vi "Ocean Optics 2000 4000 Process Spectrum.vi"() -> ()   [LabVIEW 2021]
doc: "Demonstrates measuring and processing the spectra and display in Absorbance, Transmission and Irradiance mode.\n\n<b>Note:</b>\nRefer to Spectrum Processing.vi for more details regarding the modes."
uses:
  <instrlib>/Ocean Optics 2000 4000/Ocean Optics 2000 4000.lvlib
panel:
  in  "Stop":bool
  out "Waveform":T1(graph)
  in  "Color Temperature (2850 K)":dbl=2850.0
  in  "Spectral Mode (0:Absorbance)":u16(ring) items=["Absorbance", "Transmission", "Irradiance"]
  in  "Read Reference":bool
  in  "Read Dark":bool
  in  "VISA resource name":refnum<visa-resource-name>
  # "(c) 2009-2016 National Instruments.  ALL RIGHTS RESERVED."
  # "To run this Example, select the spectral processing mode. Then run the VI. To read the dark spectrum, click Read Dark. Then click Read Reference to read Reference Spectrum. The processed spectrum will display on the graph. Press Stop when done."
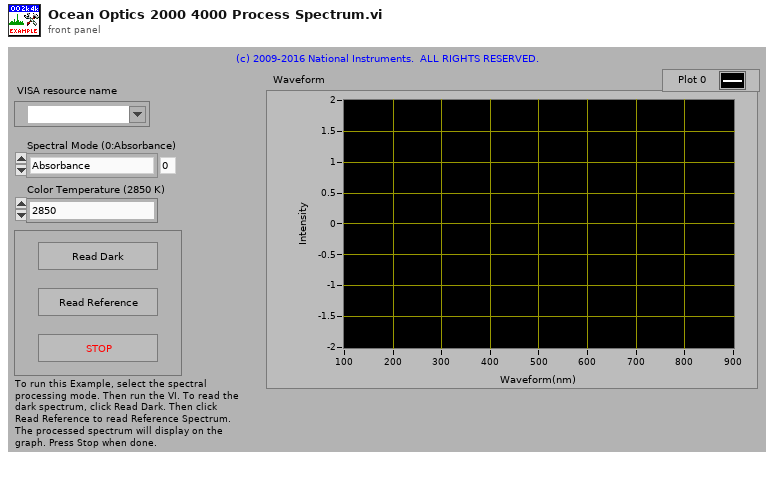
[diagram p1: front panel]
types:
  T1 = cluster{"Wavelength (nm)":dbl[], "Processed Spectrum":dbl[]}
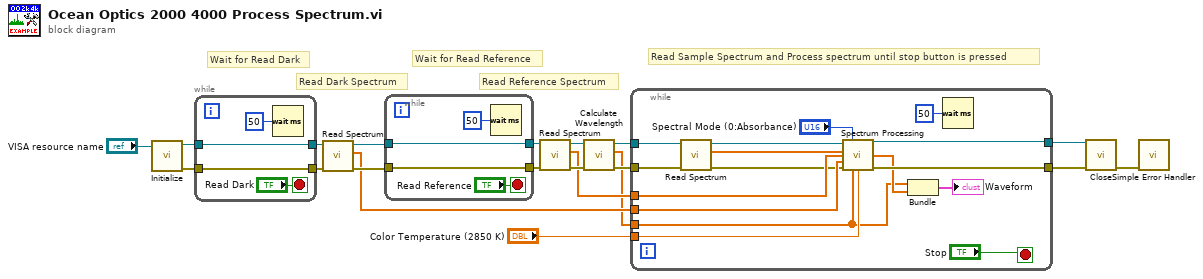
[diagram p0: block diagram]
diagram:
  # "Read Sample Spectrum and Process spectrum until stop button is pressed"
  # "Read Reference Spectrum"
  # "Read Dark Spectrum"
  # "Wait for Read Reference"
  # "Wait for Read Dark"
  n1 = call <instrlib>:"Initialize.vi"("VISA resource name"="VISA resource name") -> ("error out"=w18:errorcluster, "VISA resource name out"=w19:refnum<visa-resource-name>)  [unwired: 2 in, 7 out]
  n2 = while {
    tunnel: [w23] -> w17
    tunnel: w19 -> [w23]
    tunnel: [w22] -> w16
    tunnel: w18 -> [w22]
    stop <- "Read Dark" stop-if-true
    n3 = Wait (ms)(milliseconds to wait=u32 50 ("millisecond multiple")) -> ()  [unwired: 1 out]
  }
  n4 = call <instrlib>:"Read Spectrum.vi"("error in (no error)"=w16, "VISA resource name"=w17) -> ("error out"=w14:errorcluster, "Spectrum by Pixel Number"=w11:dbl[], "VISA resource name out"=w15:refnum<visa-resource-name>)  [unwired: 6 in, 1 out]
  n5 = while {
    tunnel: [w27] -> w12
    tunnel: w15 -> [w27]
    tunnel: [w26] -> w13
    tunnel: w14 -> [w26]
    stop <- "Read Reference" stop-if-true
    n6 = Wait (ms)(milliseconds to wait=u32 50 ("millisecond multiple")) -> ()  [unwired: 1 out]
  }
  n7 = call <instrlib>:"Read Spectrum.vi"("error in (no error)"=w13, "VISA resource name"=w12) -> ("error out"=w9:errorcluster, "Spectrum by Pixel Number"=w8:dbl[], "VISA resource name out"=w10:refnum<visa-resource-name>)  [unwired: 6 in, 1 out]
  n8 = call <instrlib>:"Calculate Wavelength.vi"("error in (no error)"=w9, "VISA resource name"=w10) -> ("error out"=w6:errorcluster, "Wavelength (nm)"=w5:dbl[], "VISA resource name out"=w7:refnum<visa-resource-name>)  [unwired: 1 in, 6 out]
  n9 = while {
    tunnel: w11 -> [w44]
    tunnel: w8 -> [w43]
    tunnel: w7 -> [w41]
    tunnel: w6 -> [w42]
    tunnel: w5 -> [w32]
    tunnel: "Color Temperature (2850 K)" -> [w37]
    tunnel: [w36] -> w3
    tunnel: [w35] -> w2
    stop <- "Stop" stop-if-true
    n10 = call <instrlib>:"Read Spectrum.vi"("error in (no error)"=w42, "VISA resource name"=w41) -> ("error out"=w39:errorcluster, "Spectrum by Pixel Number"=w38:dbl[], "VISA resource name out"=w40:refnum<visa-resource-name>)  [unwired: 6 in, 1 out]
    n11 = call <instrlib>:"Spectrum Processing.vi"("VISA resource name"=w40, "Spectral Mode (0:Absorbance)"="Spectral Mode (0:Absorbance)", "Sample Spectrum"=w38, "Reference Spectrum"=w43, "Dark Spectrum"=w44, "error in (no error)"=w39, "Wavelength (nm)"=w32, "Color Temperature (2850 K)"=w37) -> ("VISA resource name out"=w36:refnum<visa-resource-name>, "Processed Spectrum"=w33:dbl[], "error out"=w35:errorcluster)  [unwired: 5 out]
    n12 = Bundle("Wavelength (nm)"=w32, "Processed Spectrum"=w33) -> (→"Waveform":T1)  [unwired: 1 out]
    n13 = Wait (ms)(milliseconds to wait=u32 50 ("millisecond multiple")) -> ()  [unwired: 1 out]
  }
  n14 = call <instrlib>:"Close.vi"("error in (no error)"=w2, "VISA resource name"=w3) -> ("error out"=w1:errorcluster)  [unwired: 9 out]
  n15 = call <vilib>:"Simple Error Handler.vi"("error in (no error)"=w1) -> ()  [unwired: 1 in, 8 out]
